vi "Version to String.vi"(11 "Version":T1) -> (3 "String":string)   [LabVIEW 2023, in "VIDoc Printer.lvlib" / "VIDoc Printer.lvclass"]
doc: "Converts the Version cluster into a printable String"
uses:
  VIDoc Printer.lvclass
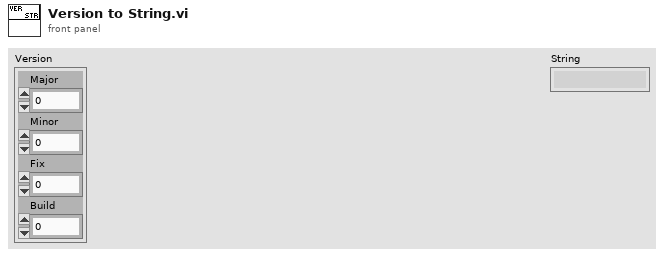
[diagram p1: front panel]
types:
  T1 = cluster{"Major":u16, "Minor":u16, "Fix":u16, "Build":u16}
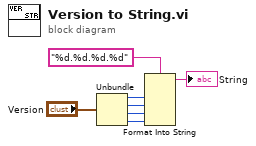
[diagram p0: block diagram]
diagram:
  n1 = Unbundle("Version") -> ("Major"=w2:u16, "Minor"=w3:u16, "Fix"=w4:u16, "Build"=w5:u16)
  n2 = Format Into String(format string="%d.%d.%d.%d", w2, w3, w4, w5) -> (resulting string=→"String":string)  [unwired: 2 in, 1 out]
